vi "Part 1.vi"(11 "Input":string) -> (3 "Output":i64)   [LabVIEW 2021]
uses:
  <userlib>/_OpenG.lib/string/string.llb/Convert EOLs (String)__ogtk.vi
panel:
  out "Antenna positions":map{string, cluster{"Row":i32, "Col":i32}[]}(c390)
  out "Map":string[][](array[string])
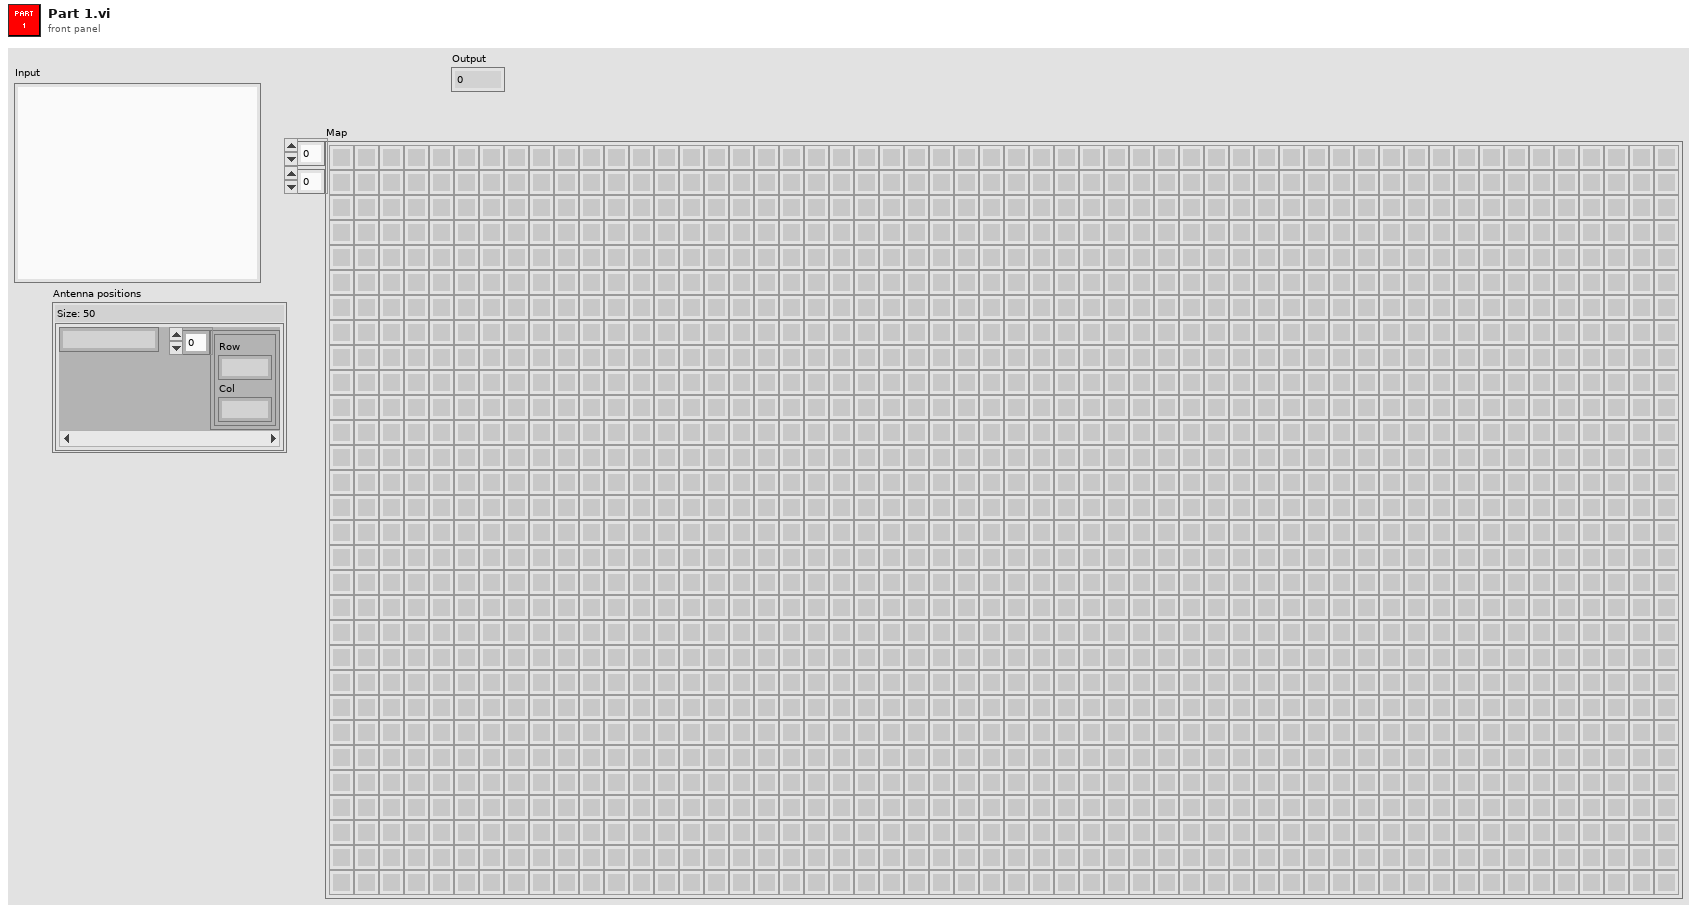
[diagram p1: front panel]
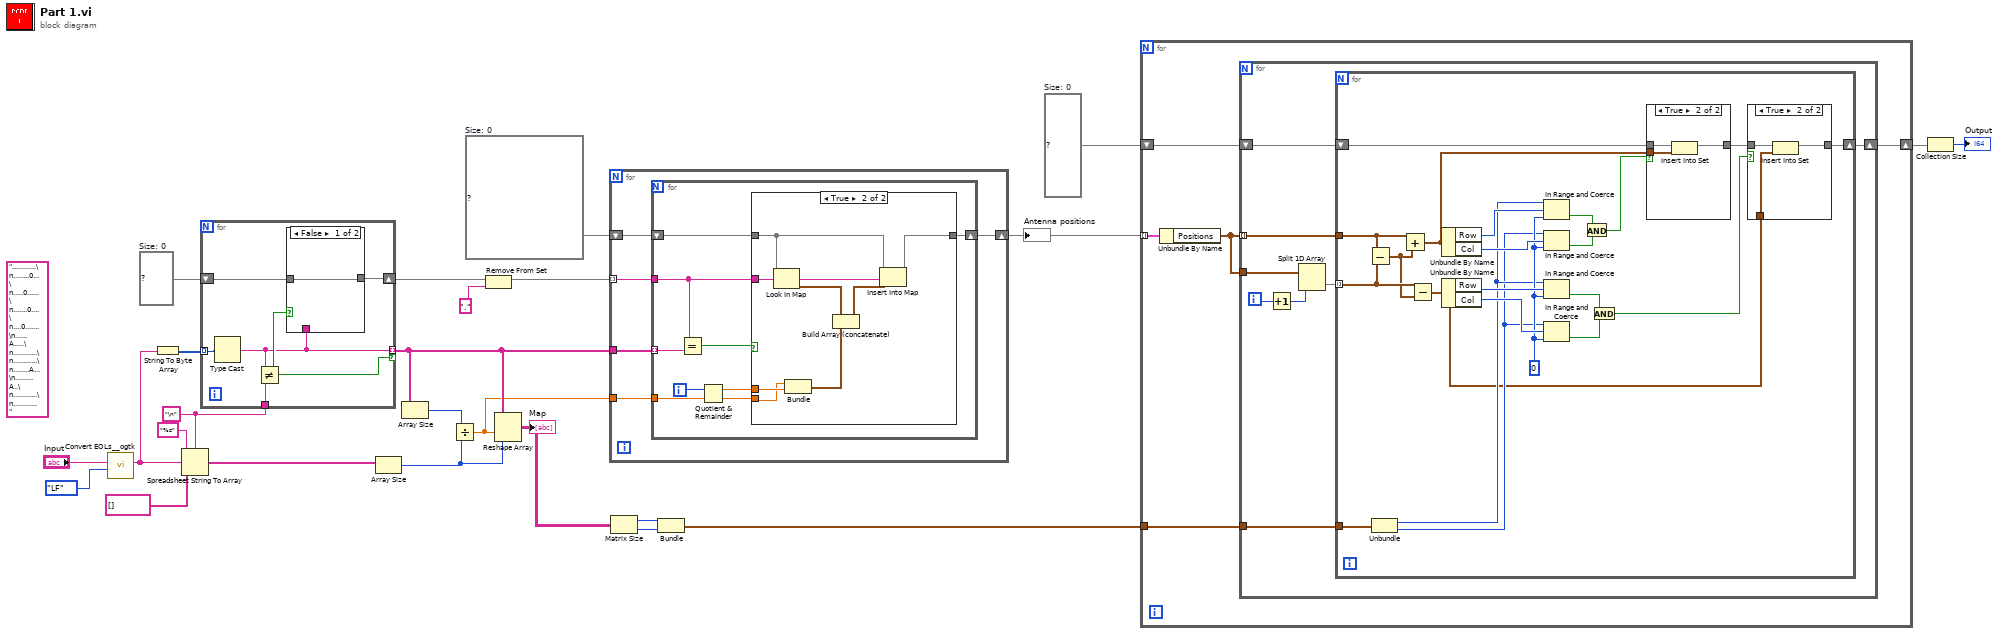
[diagram p0: block diagram]
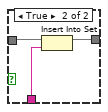
[diagram p5: hidden frame]
diagram:
  (unwired) "............\n........0...\n.....0......\n.......0....\n....0.......\n......A.....\n............\n............\n........A...\n.........A..\n............\n............"
  w8 = set{cluster{"Row":i32, "Col":i32}} {}  # Size: 0
  w14 = map{string, cluster{"Row":i32, "Col":i32}[]} {}  # Size: 0
  w16 = set{string} {}  # Size: 0
  w17 = "\n" ("delimiter (Tab)")
  n1 = call-poly <userlib>:"Convert EOLs__ogtk.vi"("Convert to:"=enum16{"CR", "LF", "CRLF"}."LF", "String in"="Input") -> ("String out"=w22:string)  [unwired: 9 in]
  n2 = String To Byte Array(string=w22) -> (unsigned byte array=w21:u8[])
  n3 = Spreadsheet String To Array(delimiter (Tab)=w17, format string="%s", spreadsheet string=w22, array type (2D Dbl)=string[] []) -> (array=w20:string[])
  n4 = for {
    tunnel: w21 -> [w31] mode=indexing
    tunnel: [w26] -> w13 mode=indexing if=w29
    tunnel: w17 -> [w30]
    shift-right: [w27] -> w15
    shift-left: w16 -> [w28]
    n5 = Type Cast(x=w31) -> (*(type *) &x=w26:string)  [unwired: 1 in]
    n6 = Not Equal?(x=w26, y=w30) -> (x != y?=w29:bool)
    n7 = case shown="False" w29 {
      tunnel: w28 -> [w32 w35]
      tunnel: [w32 w34] -> w27
      tunnel: w26 -> [_ w33]
      frame False {
      }
      frame True {
        n8 = Insert Into Set(10:w33, 11:w35) -> (3:w34:set{string})  [unwired: 1 out]
      }
    }
  }
  n9 = Array Size(array=w20) -> (size(s)=w19:i32)
  n10 = Array Size(array=w13) -> (size(s)=w18:i32)
  n11 = Divide(x=w18, y=w19) -> (x/y=w12:dbl)
  n12 = Remove From Set(10:".", 11:w15) -> (3:w11:set{string})  [unwired: 1 out]
  n13 = Reshape Array(w13, w12, w19) -> (w5:string[][])
  "Map" <- w5
  n14 = for {
    tunnel: w11 -> [w38] mode=indexing
    shift-right: [w36] -> w9
    shift-left: w14 -> [w37]
    tunnel: w13 -> [w40]
    tunnel: w12 -> [w39]
    n15 = for {
      tunnel: w40 -> [w47] mode=indexing
      tunnel: w39 -> [w48]
      tunnel: w38 -> [w43]
      shift-right: [w44] -> w36
      shift-left: w37 -> [w45]
      i -> [w49]
      n16 = Equal?(x=w43, y=w47) -> (x = y?=w46:bool)
      n17 = Quotient & Remainder(x=w49, y=w48) -> (x-y*floor(x/y)=w42:dbl, floor(x/y)=w41:dbl)
      n18 = case shown="True" w46 {
        tunnel: w45 -> [w50 w58]
        tunnel: [w50 w56] -> w44
        tunnel: w43 -> [_ w57]
        tunnel: w42 -> [_ w52]
        tunnel: w41 -> [_ w51]
        frame False {
        }
        frame True {
          n19 = Look In Map(map=w58, key=w57) -> (value=w55:cluster{"Row":i32, "Col":i32}[])  [unwired: 1 in, 1 out]
          n20 = Bundle(w51, w52) -> (w54:cluster{dbl, dbl})  [unwired: 1 in]
          n21 = Build Array (concatenate)(w55, w54) -> (w53:cluster{"Row":dbl, "Col":dbl}[])
          n22 = Insert Into Map(map in=w58, key=w57, value=w53) -> (map out=w56:map{string, cluster{"Row":i32, "Col":i32}[]})  [unwired: 2 out]
        }
      }
    }
  }
  "Antenna positions" <- w9
  n23 = Matrix Size(0:w5) -> (1:w3:i32, 2:w4:i32)
  n24 = Bundle("number of columns"=w3, "matrix"=w4) -> (w2:cluster{"number of columns":i32, "matrix":i32})  [unwired: 1 in]
  n25 = for {
    tunnel: w9 -> [w63] mode=indexing
    shift-right: [w60] -> w7
    shift-left: w8 -> [w61]
    tunnel: w2 -> [w59]
    n26 = Unbundle By Name(w63) -> ("Positions"=w62:cluster{"Row":i32, "Col":i32}[])
    n27 = for {
      tunnel: w62 -> [w68] mode=indexing
      tunnel: w62 -> [w71]
      shift-right: [w65] -> w60
      shift-left: w61 -> [w66]
      tunnel: w59 -> [w64]
      i -> [w70]
      n28 = Increment(x=w70) -> (x+1=w69:i32)
      n29 = Split 1D Array(array=w71, index=w69) -> (second subarray=w67:cluster{"Row":i32, "Col":i32}[])  [unwired: 1 out]
      n30 = for {
        tunnel: w68 -> [w93]
        tunnel: w67 -> [w92] mode=indexing
        shift-right: [w88] -> w65
        shift-left: w66 -> [w90]
        tunnel: w64 -> [w87]
        w82 = 0
        n31 = Subtract(x=w93, y=w92) -> (x-y=w91:cluster{"Row":i32, "Col":i32})
        n32 = Unbundle(w87) -> ("number of columns"=w81:i32, "matrix"=w80:i32)
        n33 = Add(x=w93, y=w91) -> (x+y=w73:cluster{"Row":i32, "Col":i32})
        n34 = Subtract(x=w92, y=w91) -> (x-y=w72:cluster{"Row":i32, "Col":i32})
        n35 = Unbundle By Name(w73) -> ("Row"=w86:i32, "Col"=w85:i32)
        n36 = Unbundle By Name(w72) -> ("Row"=w84:i32, "Col"=w83:i32)
        n37 = In Range and Coerce(upper limit=w81, x=w86, lower limit=w82) -> (In Range?=w78:bool)  [unwired: 1 out]
        n38 = In Range and Coerce(upper limit=w80, x=w85, lower limit=w82) -> (In Range?=w79:bool)  [unwired: 1 out]
        n39 = In Range and Coerce(upper limit=w81, x=w84, lower limit=w82) -> (In Range?=w75:bool)  [unwired: 1 out]
        n40 = In Range and Coerce(upper limit=w80, x=w83, lower limit=w82) -> (In Range?=w76:bool)  [unwired: 1 out]
        n41 = And(x=w78, y=w79) -> (x .and. y?=w77:bool)
        n42 = And(x=w75, y=w76) -> (x .and. y?=w74:bool)
        n43 = case shown="True" w77 {
          tunnel: w90 -> [w98 w101]
          tunnel: [w98 w100] -> w89
          tunnel: w73 -> [_ w99]
          frame False {
          }
          frame True {
            n44 = Insert Into Set(10:w99, 11:w101) -> (3:w100:set{cluster{"Row":i32, "Col":i32}})  [unwired: 1 out]
          }
        }
        n45 = case shown="True" w74 {
          tunnel: w89 -> [w94 w97]
          tunnel: [w94 w96] -> w88
          tunnel: w72 -> [_ w95]
          frame False {
          }
          frame True {
            n46 = Insert Into Set(10:w95, 11:w97) -> (3:w96:set{cluster{"Row":i32, "Col":i32}})  [unwired: 1 out]
          }
        }
      }
    }
  }
  n47 = Collection Size(1:w7) -> (0:→"Output":i32)
